vi "LEDCenter.vi"(0 "f":dbl) -> ()   [LabVIEW 2015]
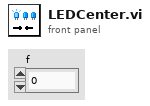
[diagram p1: front panel]
types:
  T1 = typedef "WPI_AOChannelDevRef.ctl" = cluster{"DevStatus":errorcluster, "AO Channel":T2}
  T2 = typedef "WPI_AnalogOutputChannel.ctl" = enum8{"AO MXP 0", "AO MXP 1", "Invalid"}
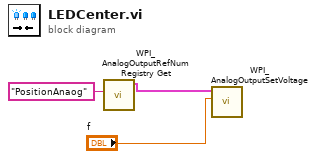
[diagram p0: block diagram]
diagram:
  n1 = call <vilib>:"WPI_AnalogOutputRefNum Registry Get.vi"("refnum name"="PositionAnaog") -> ("AODeviceRef"=w2:T1)  [unwired: 9 in, 1 out]
  n2 = call <vilib>:"WPI_AnalogOutputSetVoltage.vi"("Voltage"="f", "AODeviceRef"=w2) -> ()  [unwired: 8 in, 2 out]
